vi "ID2Target.vi"(0 "UniqueID":string) -> (4 "Target Parameters":string, 15 "Indexes":i32[](array[numeric]))   [LabVIEW 2013]
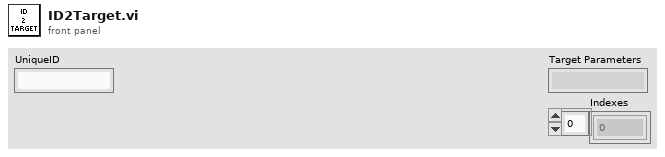
[diagram p1: front panel]
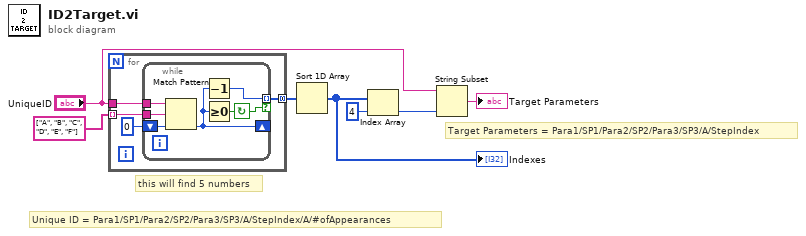
[diagram p0: block diagram]
diagram:
  # "Target Parameters = Para1/SP1/Para2/SP2/Para3/SP3/A/StepIndex"
  # "this will find 5 numbers"
  # "Unique ID = Para1/SP1/Para2/SP2/Para3/SP3/A/StepIndex/A/#ofAppearances"
  n1 = for {
    tunnel: "UniqueID" -> [w11]
    tunnel: string[] ["A", "B", "C", "D", "E", "F"] -> [w10] mode=indexing
    tunnel: [w8] -> w7 mode=concatenating
    n2 = while {
      tunnel: w11 -> [w17]
      tunnel: w10 -> [w16]
      tunnel: [w12] -> w8 mode=indexing if=w14
      shift-right: [w13] -> _
      shift-left: 0 ("offset past match") -> [w15]
      stop <- w14 continue-if-true
      n3 = Match Pattern(string=w17, regular expression=w16, offset (0)=w15) -> (offset past match=w13:i32)  [unwired: 3 out]
      n4 = Decrement(x=w13) -> (x-1=w12:i32)
      n5 = Greater Or Equal To 0?(x=w13) -> (x >= 0?=w14:bool)
    }
  }
  n6 = Sort 1D Array(array=w7) -> (sorted array=w2:i32[])
  "Indexes" <- w2
  n7 = Index Array(array=w2, index=4) -> (element=w1:i32)
  n8 = String Subset(string="UniqueID", length (rest)=w1) -> (substring=→"Target Parameters":string)  [unwired: 1 in]
